vi "LabVIEW Complex And Operations.vi"(11 "X size":i32=16384) -> (3 "LabVIEW Time":dbl)   [LabVIEW 2020]
uses:
  <vilib>/Analysis/NI_AALBase.lvlib
panel:
  in  "num_loop":i32=6
  out "max value 2":csg
  out "max value":csg
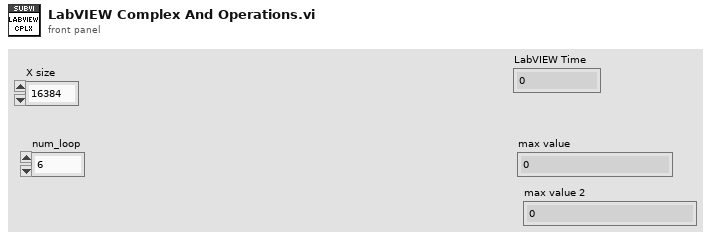
[diagram p1: front panel]
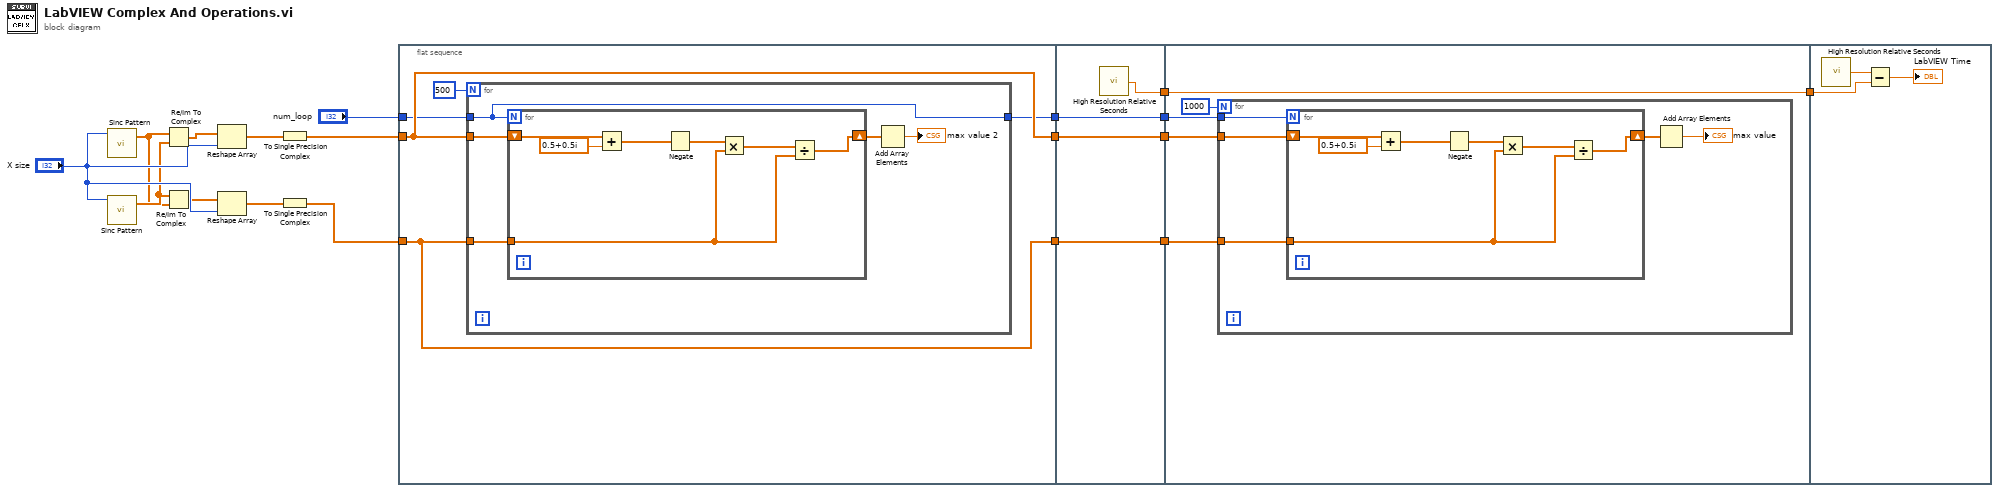
[diagram p0: block diagram]
diagram:
  n1 = call <vilib>:"Sinc Pattern.vi"("samples"="X size") -> ("Sinc Pattern"=w9:dbl[])  [unwired: 3 in, 1 out]
  n2 = call <vilib>:"Sinc Pattern.vi"("samples"="X size") -> ("Sinc Pattern"=w10:dbl[])  [unwired: 3 in, 1 out]
  n3 = Re/Im To Complex(1:w10, 2:w9) -> (0:w11:cdb[])
  n4 = Re/Im To Complex(1:w9, 2:w10) -> (0:w8:cdb[])
  n5 = Reshape Array(w11, "X size") -> (w7:cdb[])
  n6 = Reshape Array(w8, "X size") -> (w6:cdb[])
  n7 = To Single Precision Complex(1:w7) -> (0:w5:csg[])
  n8 = To Single Precision Complex(1:w6) -> (0:w4:csg[])
  n9 = flat-sequence {
    tunnel: w4 -> [w21]
    tunnel: w5 -> [w22]
    tunnel: [w22] -> w14
    tunnel: [w21] -> w13
    tunnel: "num_loop" -> [w20]
    tunnel: [w19] -> w1
    tunnel: [w39] -> w18
    tunnel: [w38] -> w16
    tunnel: [w37] -> w15
    tunnel: w14 -> [w38]
    tunnel: w13 -> [w37]
    tunnel: [w36] -> w2
    tunnel: w1 -> [w36]
    tunnel: w18 -> [w44]
    tunnel: [w44] -> w17
    tunnel: w16 -> [w43]
    tunnel: w15 -> [w42]
    tunnel: w2 -> [w40]
    tunnel: w17 -> [w58]
    frame #0 {
      n10 = for {
        N: 500 -> [_]
        tunnel: w22 -> [w28]
        tunnel: w21 -> [w27]
        tunnel: w20 -> [w24]
        tunnel: [w24] -> w19
        n11 = for {
          N: w24 -> [_]
          tunnel: w27 -> [w32]
          shift-right: [w30] -> w26
          shift-left: w28 -> [w33]
          n12 = Add(x=w33, y=csg 0.5+0.5i) -> (x+y=w29:csg[])
          n13 = Negate(x=w29) -> (-x=w34:csg[])
          n14 = Multiply(x=w34, y=w32) -> (x*y=w35:csg[])
          n15 = Divide(x=w35, y=w32) -> (x/y=w30:csg[])
        }
        n16 = Add Array Elements(numeric array=w26) -> (sum=→"max value 2":csg)
      }
    }
    frame #1 {
      n17 = call <vilib>:"High Resolution Relative Seconds.vi"() -> ("relative seconds"=w39:dbl)
    }
    frame #2 {
      n18 = for {
        N: 1000 -> [_]
        tunnel: w43 -> [w48]
        tunnel: w42 -> [w47]
        tunnel: w40 -> [w45]
        n19 = for {
          N: w45 -> [_]
          tunnel: w47 -> [w53]
          shift-right: [w51] -> w49
          shift-left: w48 -> [w54]
          n20 = Add(x=w54, y=csg 0.5+0.5i) -> (x+y=w50:csg[])
          n21 = Negate(x=w50) -> (-x=w55:csg[])
          n22 = Multiply(x=w55, y=w53) -> (x*y=w56:csg[])
          n23 = Divide(x=w56, y=w53) -> (x/y=w51:csg[])
        }
        n24 = Add Array Elements(numeric array=w49) -> (sum=→"max value":csg)
      }
    }
    frame #3 {
      n25 = call <vilib>:"High Resolution Relative Seconds.vi"() -> ("relative seconds"=w59:dbl)
      n26 = Subtract(x=w59, y=w58) -> (x-y=→"LabVIEW Time":dbl)
    }
  }
